vi "HEWH Temperature Filter (Thermal).vi"(0 "HEWH Data":T2, 1 "LV Program":T1, 11 "error in (no error)":errorcluster) -> (4 "HEWH Data Out":T2, 15 "error out":errorcluster)   [LabVIEW 2023]
uses:
  Type Definitions/HEWH Power Data.ctl
  Utility/Save File/File Setup (Public)/Type Definition/Save File DOE LabView Program.ctl
  Utility/Save File/File Setup.lvlib
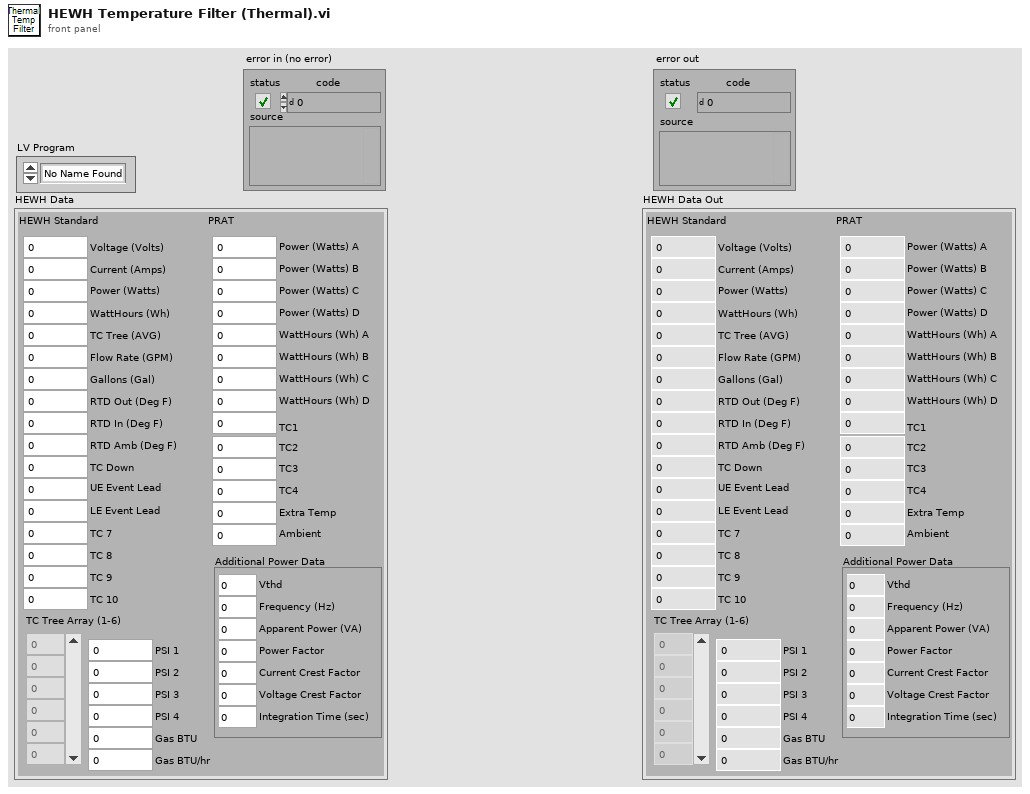
[diagram p1: front panel]
types:
  T1 = typedef "File Setup.lvlib/Save File DOE LabView Program.ctl" = enum16{"No Name Found", "DOE Stand", "Dishwasher Kitchen", "Portable Stand", "HEWH", "Dryer", "Dryer WILT", "HCC", "PRAT", "HEWH RLT", "Refrigeration", "Gas Water Heater"}
  T2 = typedef "HEWH Power Data.ctl" = cluster{"HEWH Standard":cluster{"Voltage (Volts)":dbl, "Current (Amps)":dbl, "Power (Watts)":dbl, "WattHours (Wh)":dbl, "TC Tree (AVG)":dbl, "Flow Rate (GPM)":dbl, "Gallons (Gal)":dbl, "RTD Out (Deg F)":dbl, "RTD In (Deg F)":dbl, "RTD Amb (Deg F)":dbl, "TC Down":dbl, "UE Event Lead":i32, "LE Event Lead":i32, "TC 8":dbl, "TC 9":dbl, "TC 10":dbl, "TC Tree Array (1-6)":dbl[], "TC 7":dbl, "PSI 1":dbl, "PSI 2":dbl, "PSI 3":dbl, "PSI 4":dbl, "Gas BTU":dbl, "Gas BTU/hr":dbl}, "PRAT":cluster{"Power (Watts) A":dbl, "Power (Watts) B":dbl, "Power (Watts) C":dbl, "Power (Watts) D":dbl, "TC1":dbl, "TC2":dbl, "TC3":dbl, "TC4":dbl, "WattHours (Wh) A":dbl, "WattHours (Wh) B":dbl, "WattHours (Wh) C":dbl, "WattHours (Wh) D":dbl, "Ambient":dbl, "Extra Temp":dbl}, "Additional Power Data":cluster{"Vthd":dbl, "Frequency (Hz)":dbl, "Apparent Power (VA)":dbl, "Power Factor":dbl, "Current Crest Factor":dbl, "Voltage Crest Factor":dbl, "Integration Time (sec)":dbl}}
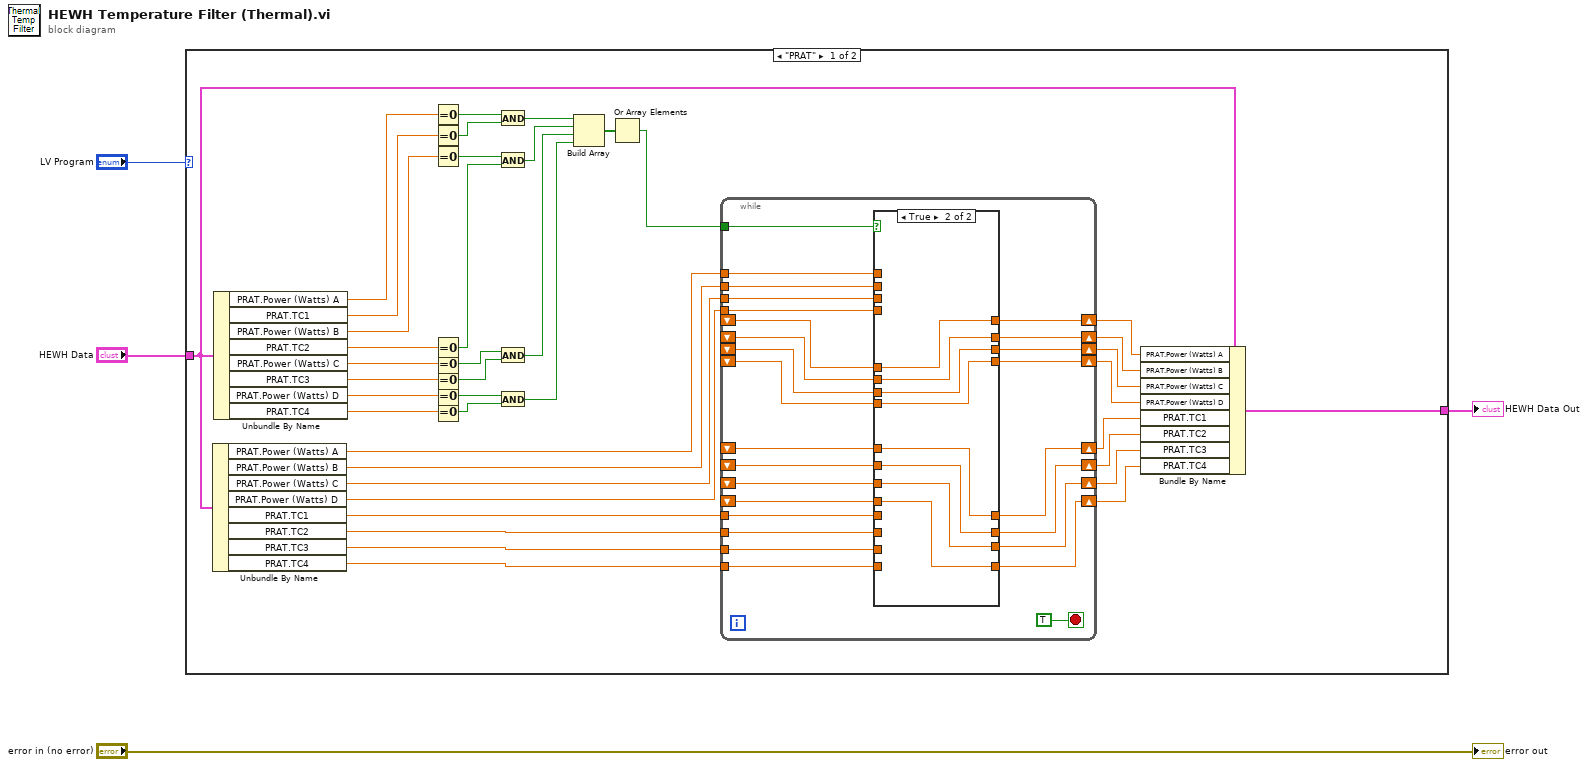
[diagram p0: block diagram]
diagram:
  n1 = case shown="\"PRAT\"" "LV Program" {
    tunnel: "HEWH Data" -> [w13 w87]
    tunnel: [w14 w87] -> w2
    frame "PRAT" {
      n2 = Unbundle By Name(w13) -> ("PRAT.Power (Watts) A"=w22:dbl, "PRAT.Power (Watts) B"=w21:dbl, "PRAT.Power (Watts) C"=w20:dbl, "PRAT.Power (Watts) D"=w19:dbl, "PRAT.TC1"=w18:dbl, "PRAT.TC2"=w17:dbl, "PRAT.TC3"=w16:dbl, "PRAT.TC4"=w15:dbl)
      n3 = Unbundle By Name(w13) -> ("PRAT.Power (Watts) A"=w44:dbl, "PRAT.TC1"=w43:dbl, "PRAT.Power (Watts) B"=w42:dbl, "PRAT.TC2"=w41:dbl, "PRAT.Power (Watts) C"=w40:dbl, "PRAT.TC3"=w39:dbl, "PRAT.Power (Watts) D"=w38:dbl, "PRAT.TC4"=w37:dbl)
      n4 = Equal To 0?(x=w44) -> (x = 0?=w36:bool)
      n5 = Equal To 0?(x=w43) -> (x = 0?=w35:bool)
      n6 = Equal To 0?(x=w42) -> (x = 0?=w34:bool)
      n7 = Equal To 0?(x=w41) -> (x = 0?=w33:bool)
      n8 = Equal To 0?(x=w40) -> (x = 0?=w32:bool)
      n9 = Equal To 0?(x=w39) -> (x = 0?=w31:bool)
      n10 = Equal To 0?(x=w38) -> (x = 0?=w30:bool)
      n11 = Equal To 0?(x=w37) -> (x = 0?=w29:bool)
      n12 = And(x=w36, y=w35) -> (x .and. y?=w28:bool)
      n13 = And(x=w34, y=w33) -> (x .and. y?=w27:bool)
      n14 = And(x=w32, y=w31) -> (x .and. y?=w26:bool)
      n15 = And(x=w30, y=w29) -> (x .and. y?=w25:bool)
      n16 = Build Array(w28, w27, w26, w25) -> (w24:bool[])
      n17 = Or Array Elements(Boolean array=w24) -> (logical OR=w23:bool)
      n18 = while {
        tunnel: w21 -> [w68]
        tunnel: w22 -> [w69]
        shift-right: [w67] -> w12
        shift-left: _ -> [w65]
        shift-right: [w66] -> w11
        shift-left: _ -> [w64]
        tunnel: w23 -> [w63]
        tunnel: w20 -> [w62]
        tunnel: w19 -> [w61]
        tunnel: w18 -> [w60]
        tunnel: w17 -> [w59]
        tunnel: w16 -> [w58]
        tunnel: w15 -> [w57]
        shift-right: [w56] -> w10
        shift-left: _ -> [w50]
        shift-right: [w55] -> w9
        shift-left: _ -> [w49]
        shift-right: [w54] -> w8
        shift-left: _ -> [w48]
        shift-right: [w53] -> w7
        shift-left: _ -> [w47]
        shift-right: [w52] -> w6
        shift-left: _ -> [w46]
        shift-right: [w51] -> w5
        shift-left: _ -> [w45]
        stop <- TRUE stop-if-true
        n19 = case shown="True" w63 {
          tunnel: w69 -> [w78 _]
          tunnel: w68 -> [w77 _]
          tunnel: [w78 w86] -> w67
          tunnel: [w77 w85] -> w66
          tunnel: w65 -> [_ w86]
          tunnel: w64 -> [_ w85]
          tunnel: w62 -> [w76 _]
          tunnel: w61 -> [w75 _]
          tunnel: w60 -> [w74 _]
          tunnel: w59 -> [w73 _]
          tunnel: w58 -> [w72 _]
          tunnel: w57 -> [w71 _]
          tunnel: [w76 w84] -> w56
          tunnel: [w75 w83] -> w55
          tunnel: [w74 w82] -> w54
          tunnel: [w73 w81] -> w53
          tunnel: [w72 w80] -> w52
          tunnel: [w71 w79] -> w51
          tunnel: w50 -> [_ w84]
          tunnel: w49 -> [_ w83]
          tunnel: w48 -> [_ w82]
          tunnel: w47 -> [_ w81]
          tunnel: w46 -> [_ w80]
          tunnel: w45 -> [_ w79]
          frame False {
          }
          frame True {
          }
        }
      }
      n20 = Bundle By Name(cluster=w13, "PRAT.Power (Watts) A"=w12, "PRAT.Power (Watts) B"=w11, "PRAT.Power (Watts) C"=w10, "PRAT.Power (Watts) D"=w9, "PRAT.TC1"=w8, "PRAT.TC2"=w7, "PRAT.TC3"=w6, "PRAT.TC4"=w5) -> (w14:T2)
    }
    frame Default {
    }
  }
  "HEWH Data Out" <- w2
  "error out" <- "error in (no error)"
